vi "Fetch External Data Log.vi"(8 "error in (no error)":errorcluster {"code" format="%.0x"}, 9 "Max Records (1)":i32=1, 10 "Channel Name (1)":string="1", 11 "VISA resource name":refnum<visa-resource-name>) -> (0 "error out":errorcluster {"code" format="%.0x"}, 2 "External Log":string, 3 "VISA resource name out":refnum<visa-resource-name>)   [LabVIEW 2010, in "Agilent N6700 Series.lvlib"]
doc: "Returns external datalog data from the instrument's buffer."
uses:
  Agilent N6700 Series.lvlib
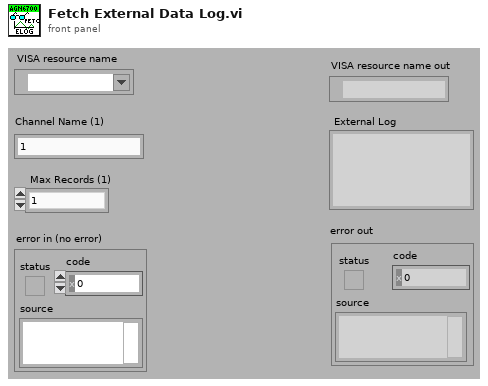
[diagram p1: front panel]
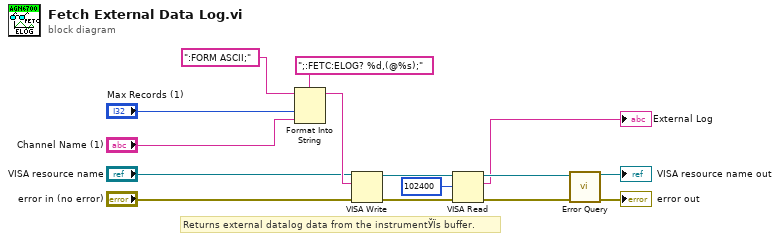
[diagram p0: block diagram]
diagram:
  # "Returns external datalog data from the instrumentЎЇs buffer."
  n1 = Format Into String(format string=";:FETC:ELOG? %d,(@%s);", initial string=":FORM ASCII;", "Max Records (1)", "Channel Name (1)") -> (resulting string=w13:string)  [unwired: 1 in, 1 out]
  n2 = VISA Write(VISA resource name="VISA resource name", write buffer=w13, error in (no error)="error in (no error)") -> (VISA resource name out=w9:refnum<visa-resource-name>, error out=w10:errorcluster)  [unwired: 1 out]
  n3 = VISA Read(VISA resource name=w9, byte count=u32 102400, error in (no error)=w10) -> (VISA resource name out=w7:refnum<visa-resource-name>, read buffer=→"External Log":string, error out=w8:errorcluster)  [unwired: 1 out]
  n4 = call "Error Query.vi"("VISA resource name"=w7, "error in (no error)"=w8) -> ("VISA resource name out"=→"VISA resource name out":refnum<visa-resource-name>, "error out"=→"error out":errorcluster)  [unwired: 10 in, 2 out]
